vi "ChromaReadReplyMsg.vi"(10 "Boolean_MsgReceiveErr?":bool, 11 "Str_ReplyIn":string) -> (0 "Clu_Result?":T1, 1 "Clu_StepParametersOut":T5, 2 "Str_MsgOut":string, 3 "Enum_ReplyMessage":T6(ring), 4 "Clu_PresetParameterOut":T4, 5 "Clu_RemoteOffsetKeylockResultOut":T2, 6 "Clu_SysSettingOut":T3)   [LabVIEW 2016]
uses:
  TypeDef/Enum_ResultCode.ctl
panel:
  out "BooleanFlag":bool
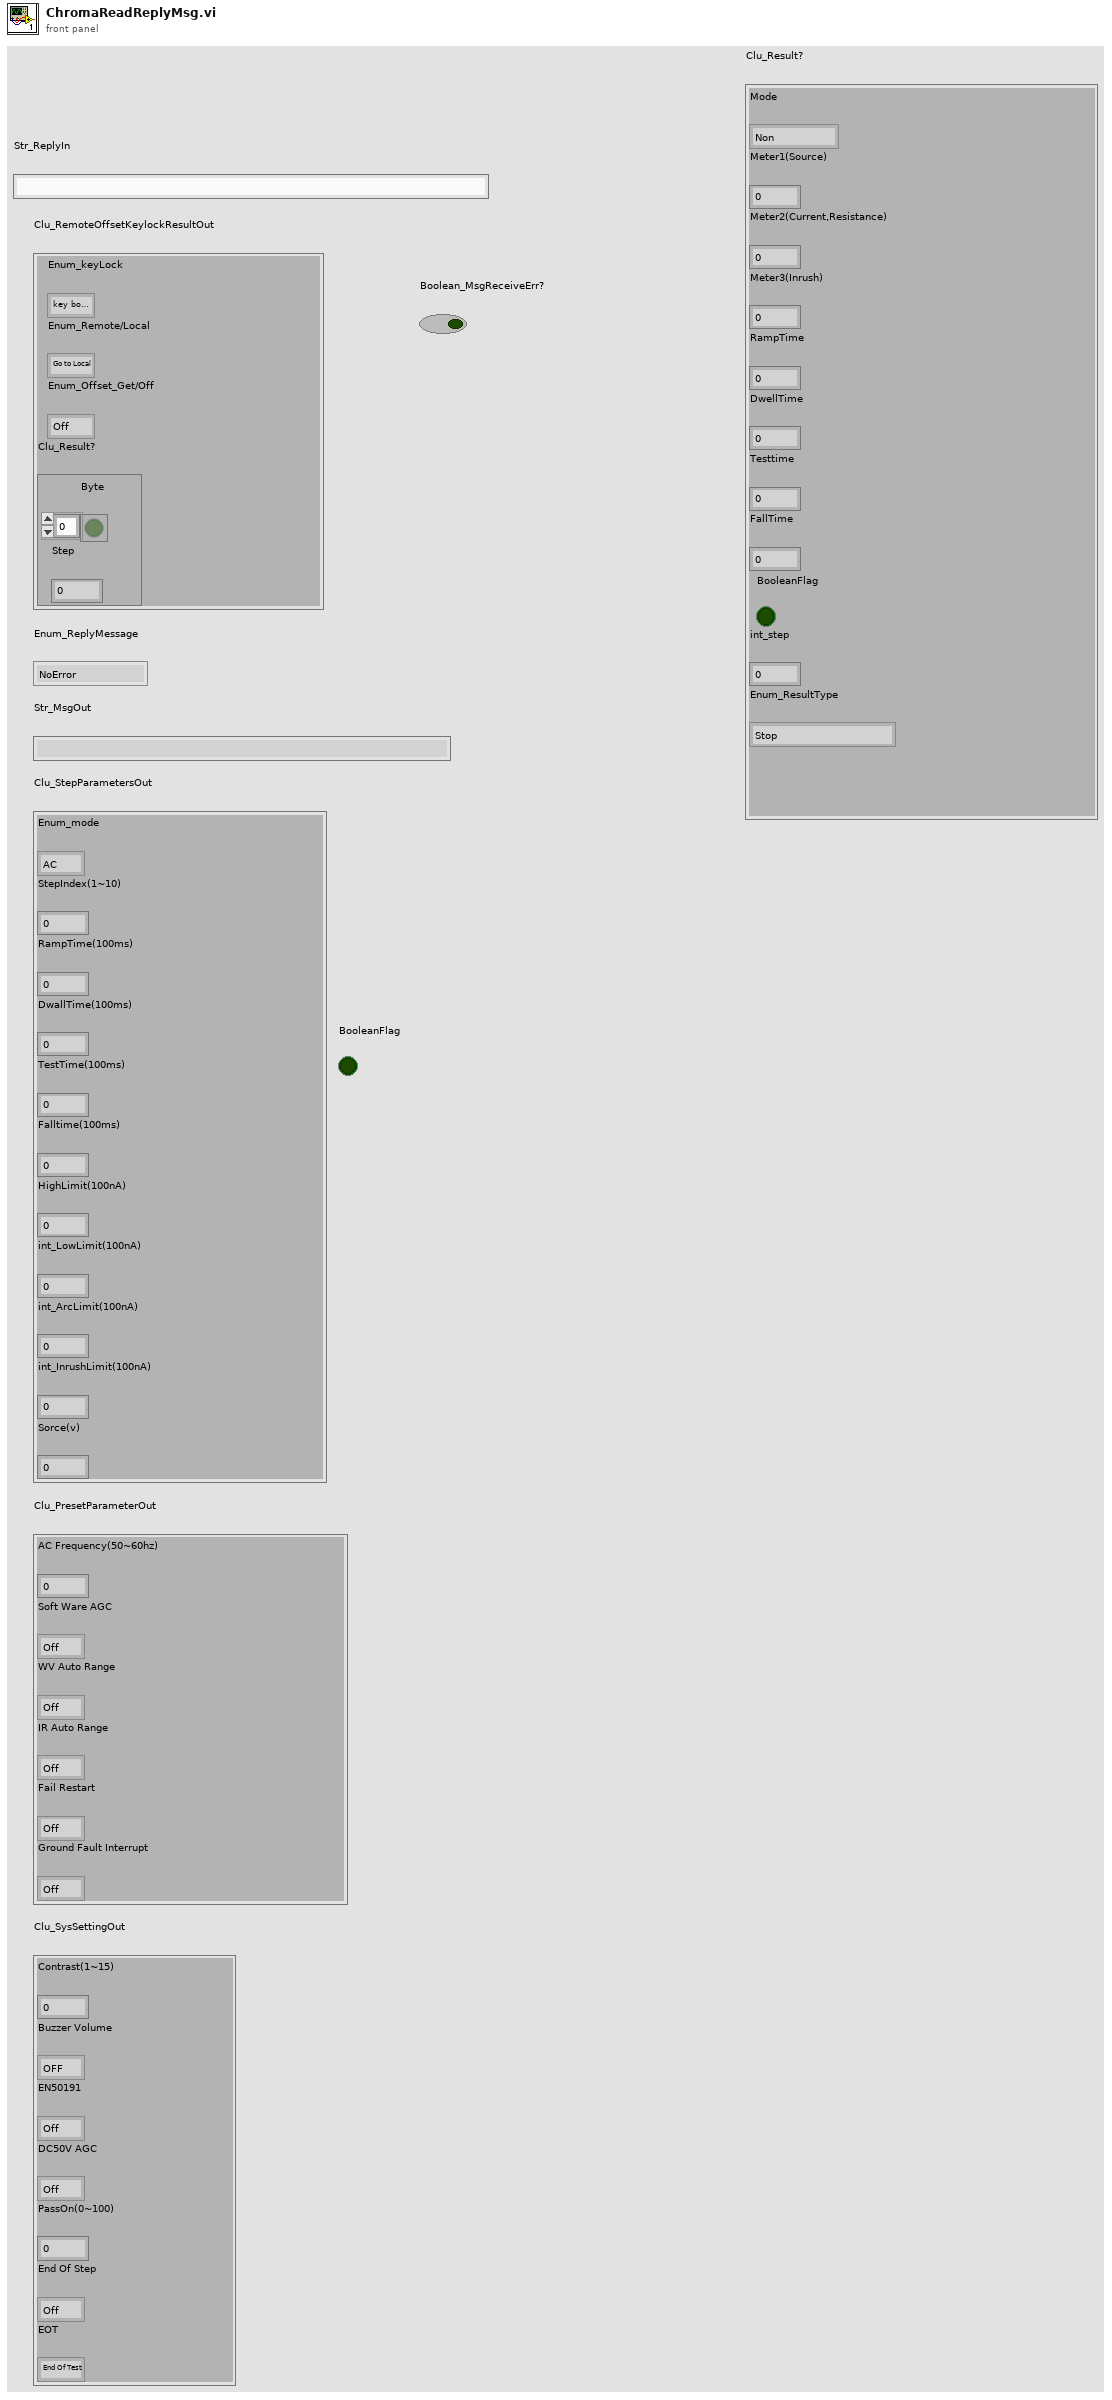
[diagram p1: front panel]
types:
  T1 = cluster{"Mode":enum8{"Non", "AC", "DC", "IR"}, "Meter1(Source)":u16, "Meter2(Current,Resistance)":u32, "Meter3(Inrush)":u32, "RampTime":u16, "DwellTime":u16, "Testtime":u16, "FallTime":u16, "BooleanFlag":bool, "int_step":u8, "Enum_ResultType":enum8{"Stop", "User Interupt", "Can not test", "Testing", "Pass", "Skipped", "GFI Tripped"}}
  T2 = cluster{"Enum_keyLock":enum8{"key board lock Off,recall key lock Off", "key board lock On,recall key lock Off", "key board lock On,recall key lock On"}, "Enum_Remote/Local":enum8{"Go to Local", "Go to Remote", "Go to Remote and Local Lockout"}, "Enum_Offset_Get/Off":enum8{"Off", "Nonuse", "Get"}, "Clu_Result?":cluster{"Byte":bool[], "Step":u8}}
  T3 = cluster{"Contrast(1~15)":u8, "Buzzer Volume":enum8{"OFF", "LOW", "Medium", "High"}, "EN50191":enum8{"Off", "On"}, "DC50V AGC":enum8{"Off", "On"}, "PassOn(0~100)":u8, "End Of Step":enum8{"Off", "On"}, "EOT":enum8{"End Of Test", "End Of Timer"}}
  T4 = cluster{"AC Frequency(50~60hz)":u8, "Soft Ware AGC":enum8{"Off", "On"}, "WV Auto Range":enum8{"Off", "On"}, "IR Auto Range":enum8{"Off", "On"}, "Fail Restart":enum8{"Off", "On"}, "Ground Fault Interrupt":enum8{"Off", "On"}}
  T5 = cluster{"Enum_mode":enum16{"AC", "DC", "IR"}, "StepIndex(1~10)":u8, "RampTime(100ms)":u16, "DwallTime(100ms)":u16, "TestTime(100ms)":u16, "Falltime(100ms)":u16, "HighLimit(100nA)":u32, "int_LowLimit(100nA)":u32, "int_ArcLimit(100nA)":u32, "int_InrushLimit(100nA)":u32, "Sorce(v)":u16}
  T6 = enum16{"NoError", "CommendError", "ParameterError"}
  T7 = enum16{"big-endian, network order", "native, host order", "little-endian"}
  T8 = typedef "Enum_ResultCode.ctl" = enum8{"Stop", "User Interupt", "Can not test", "Testing", "Pass", "Skipped", "GFI Tripped"}
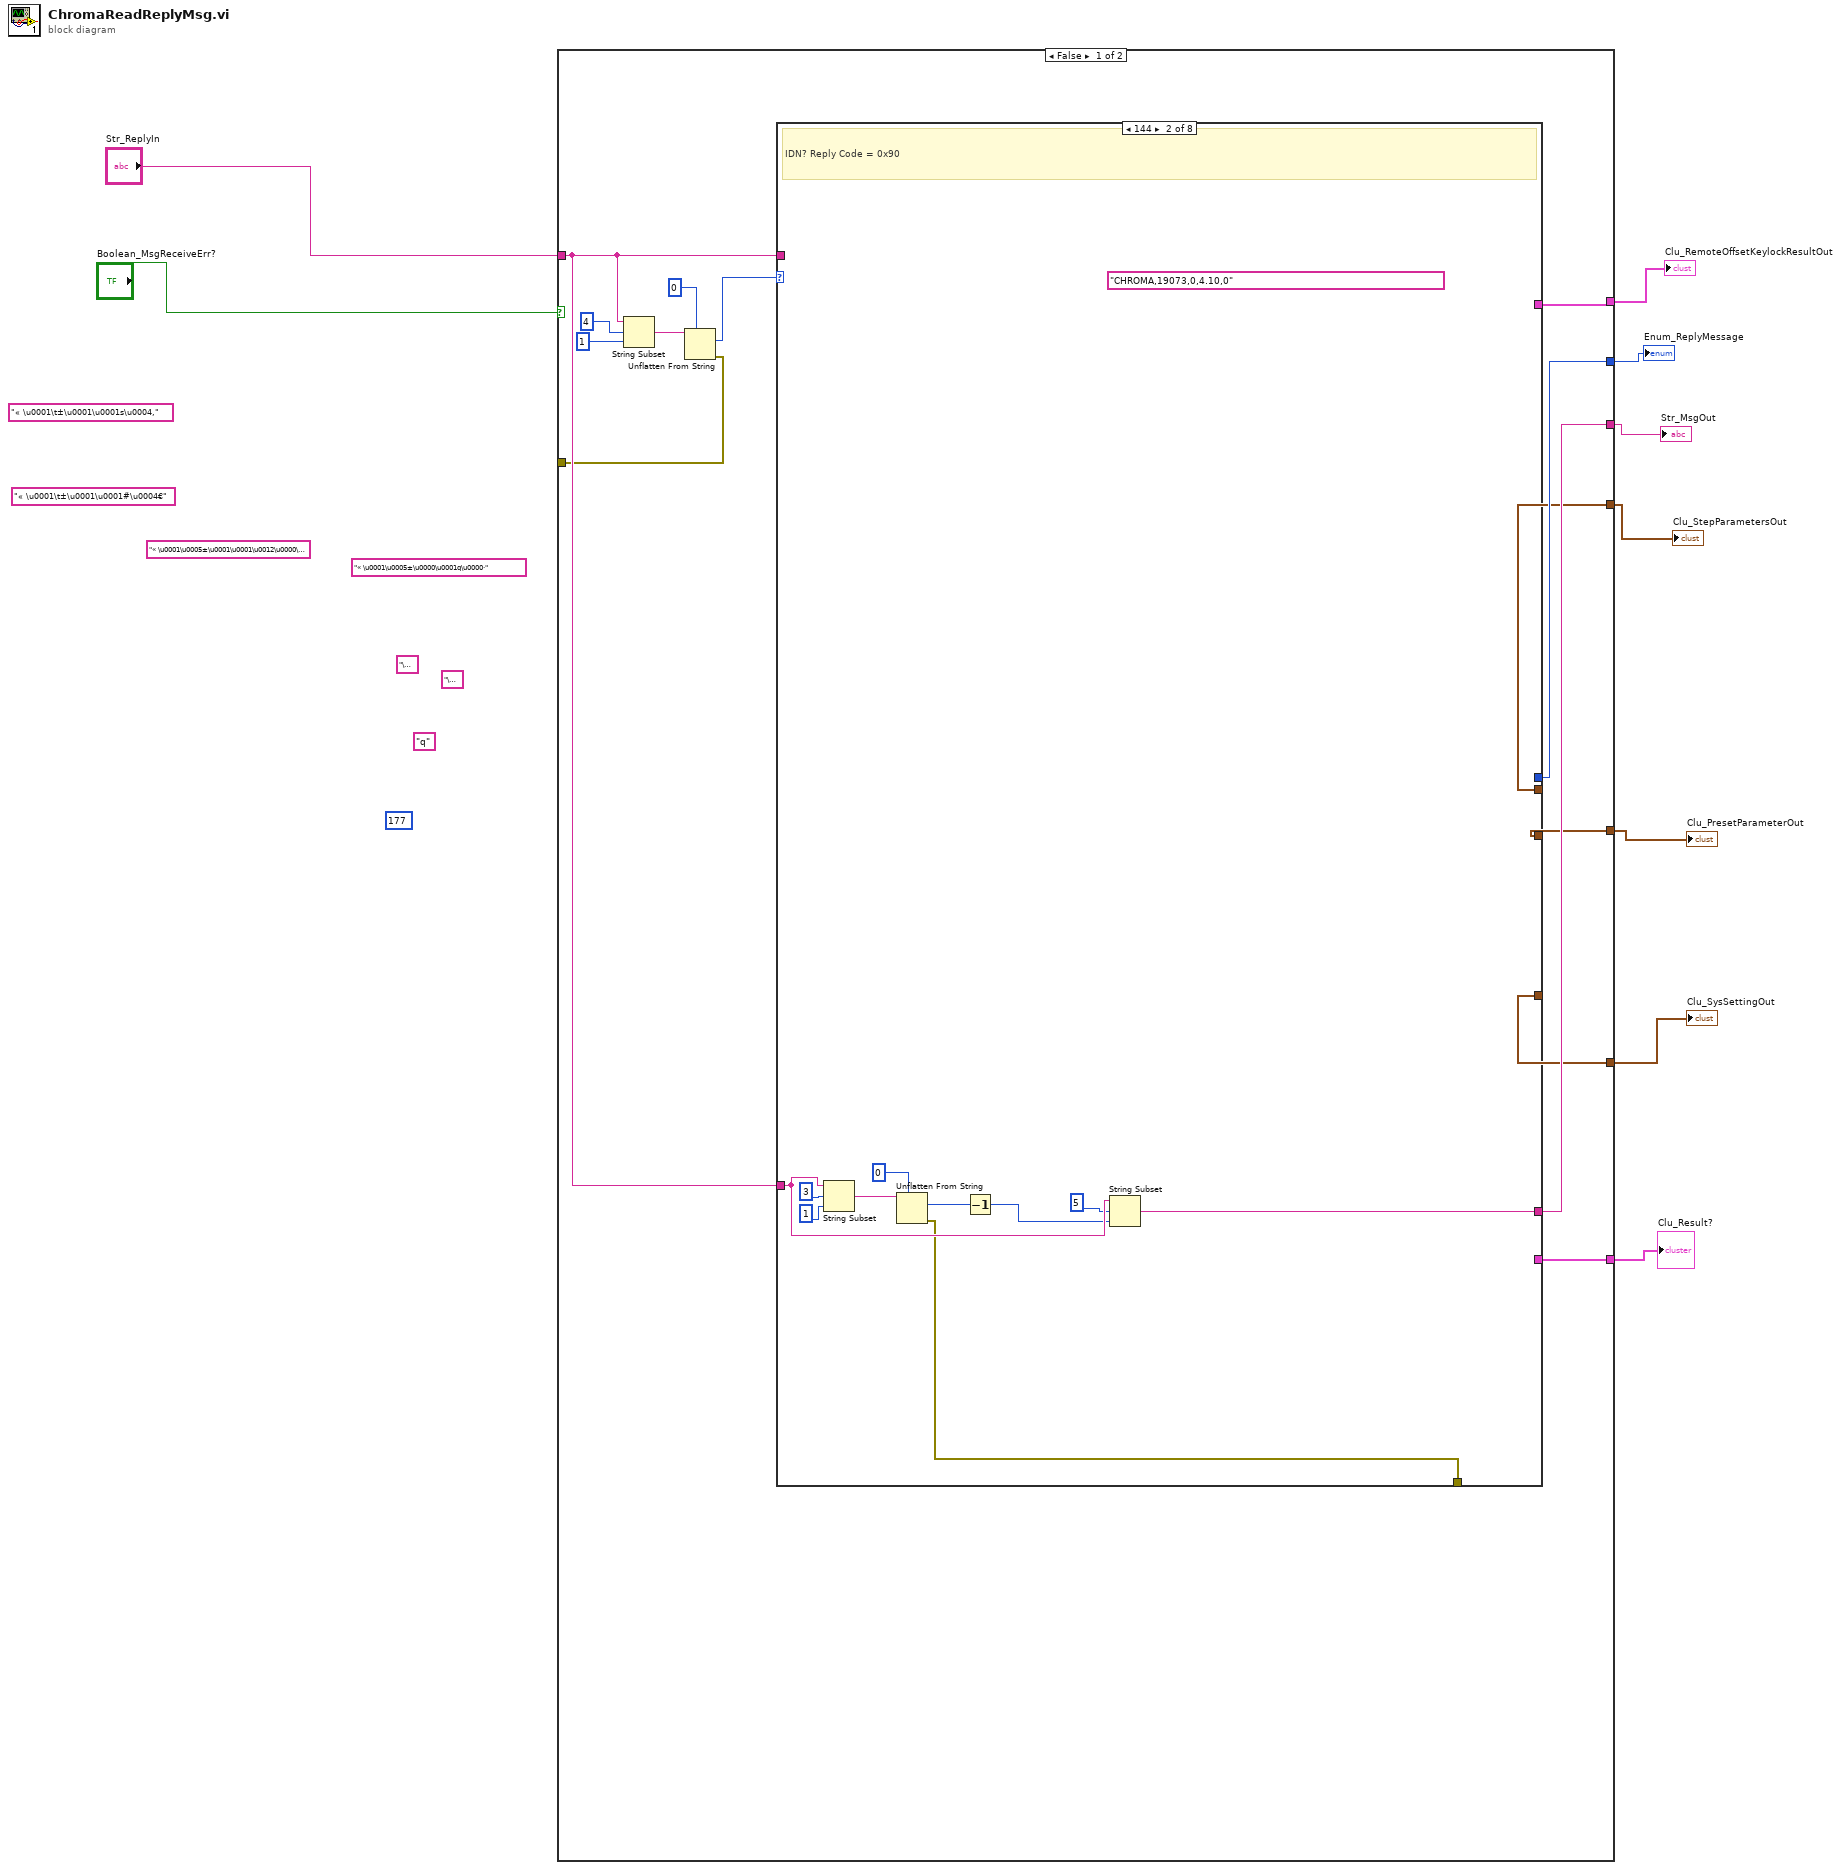
[diagram p0: block diagram]
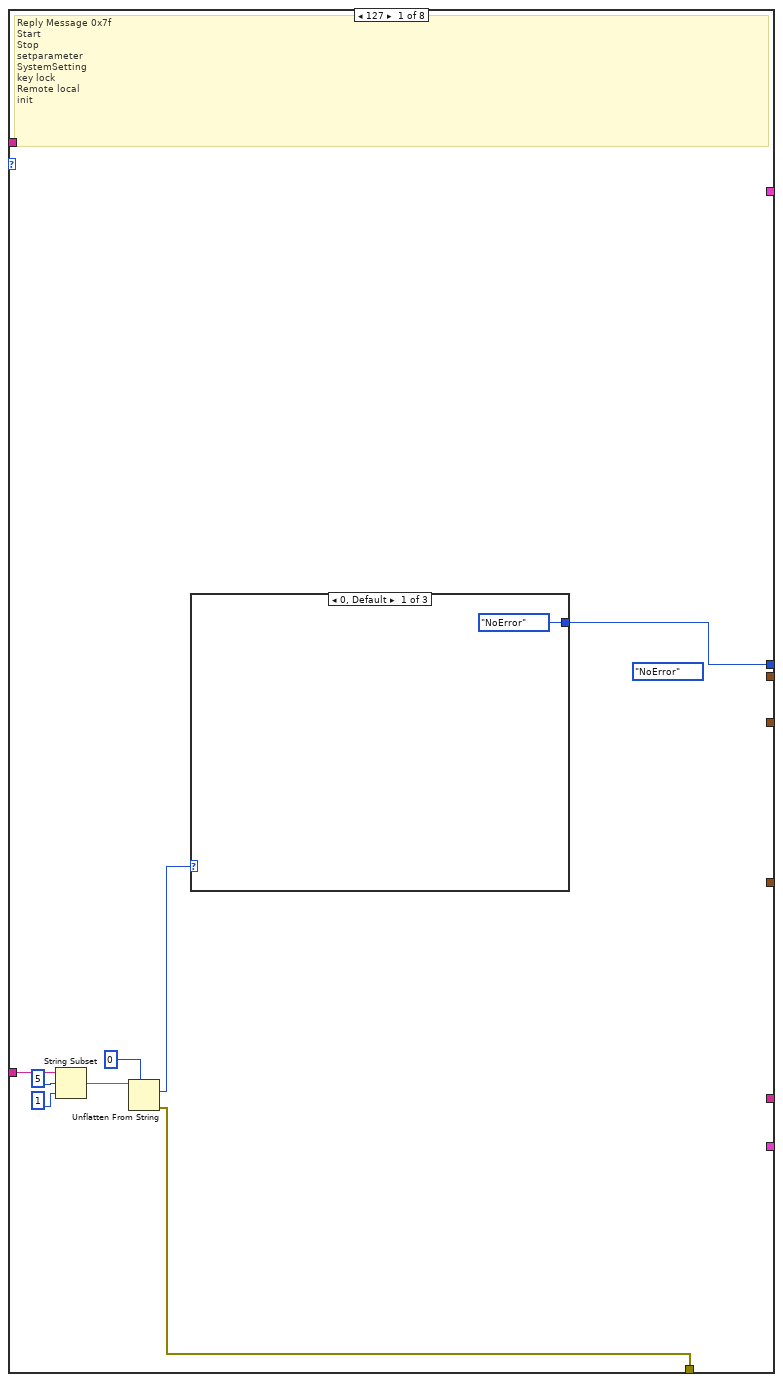
[diagram p2: hidden frame]
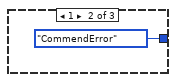
[diagram p3: hidden frame]
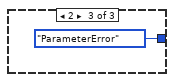
[diagram p4: hidden frame]
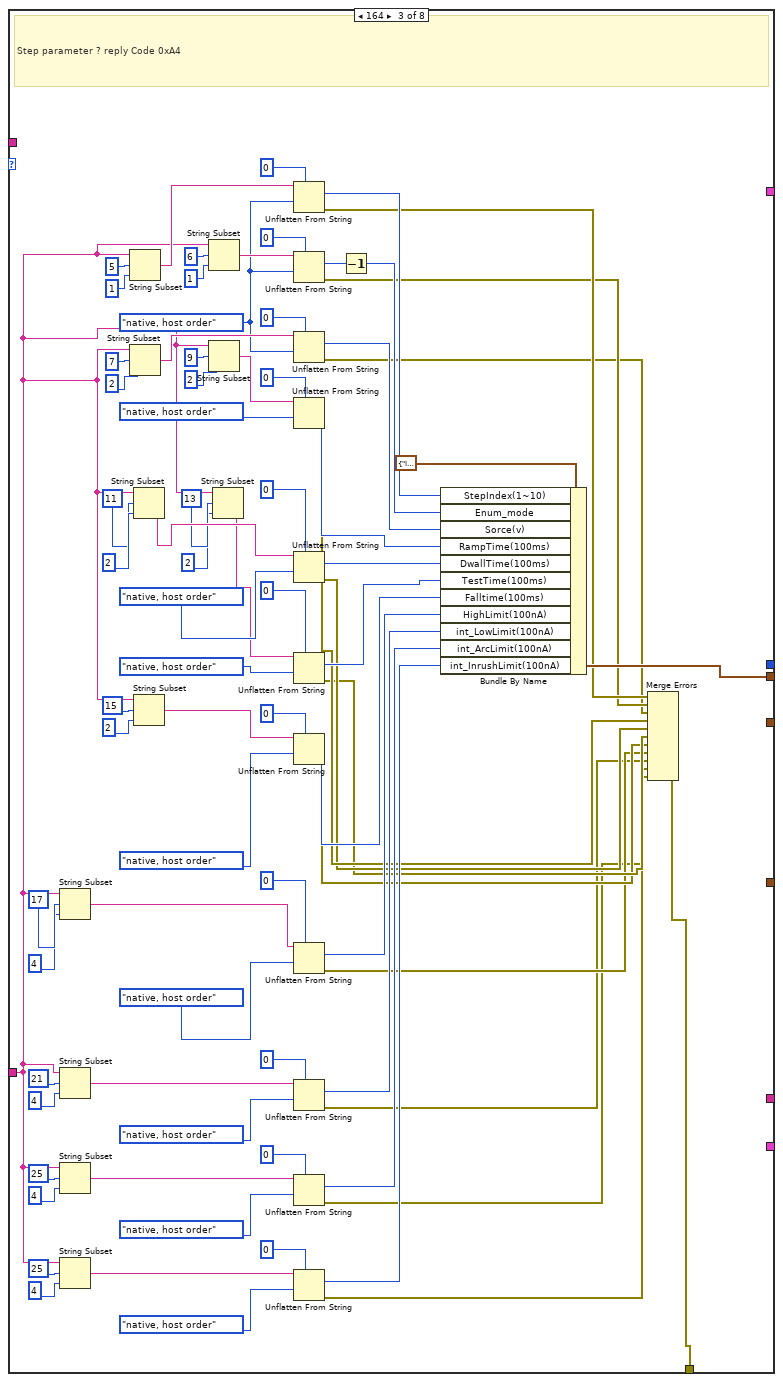
[diagram p5: hidden frame]
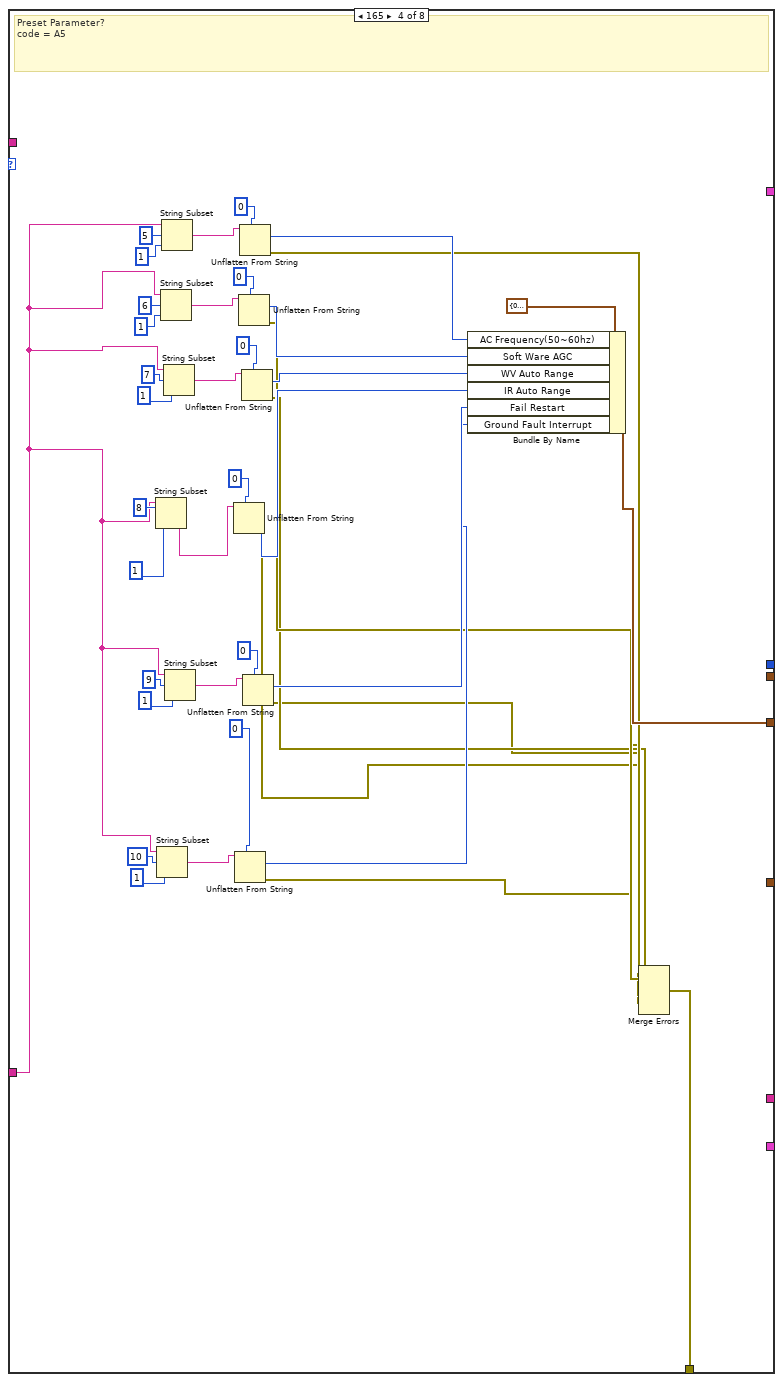
[diagram p6: hidden frame]
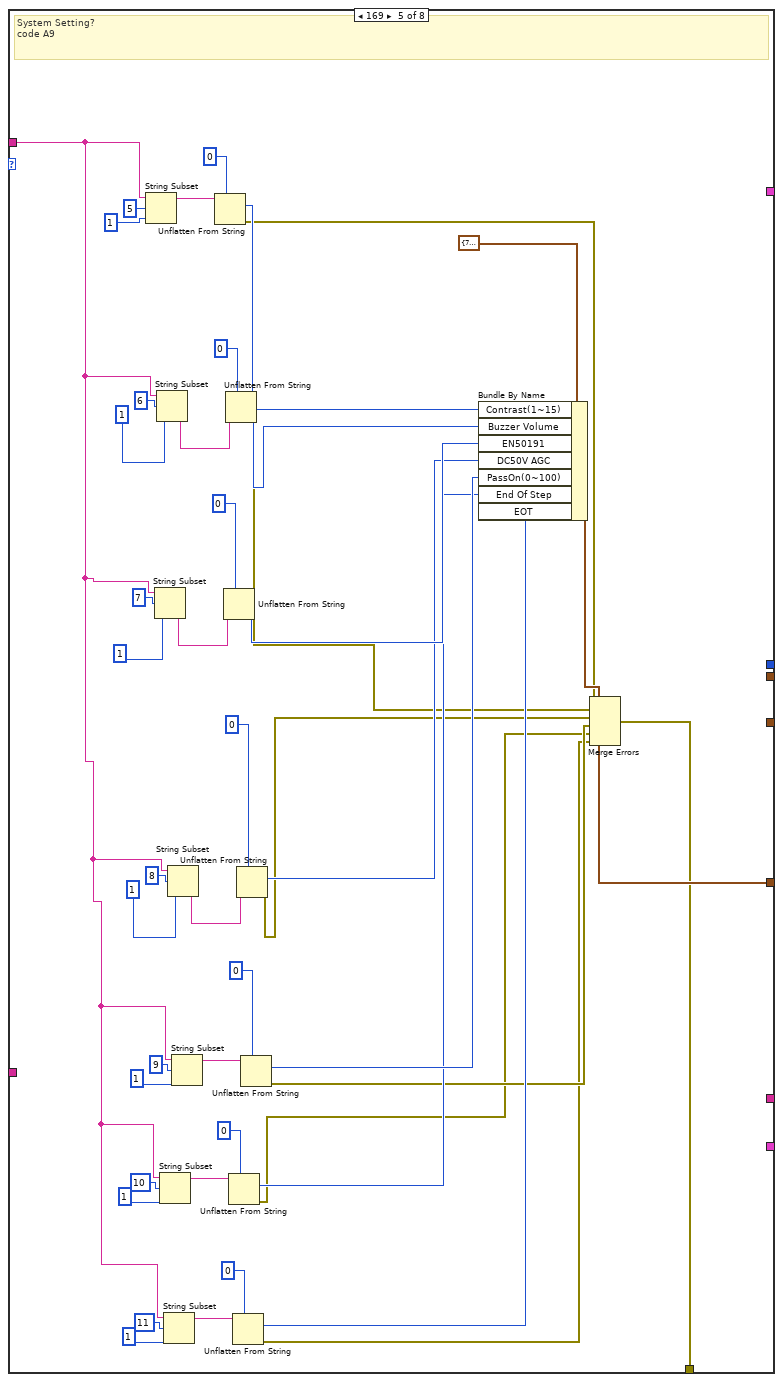
[diagram p7: hidden frame]
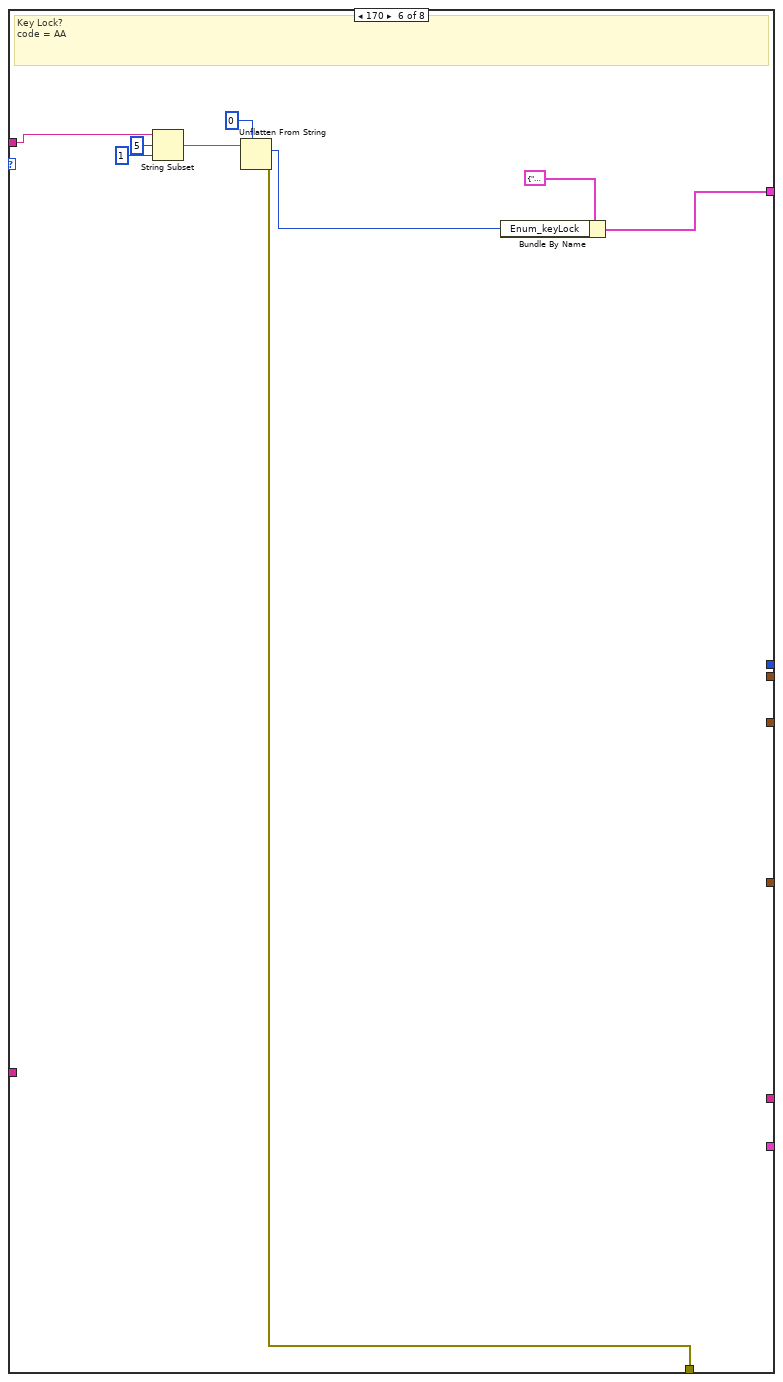
[diagram p8: hidden frame]
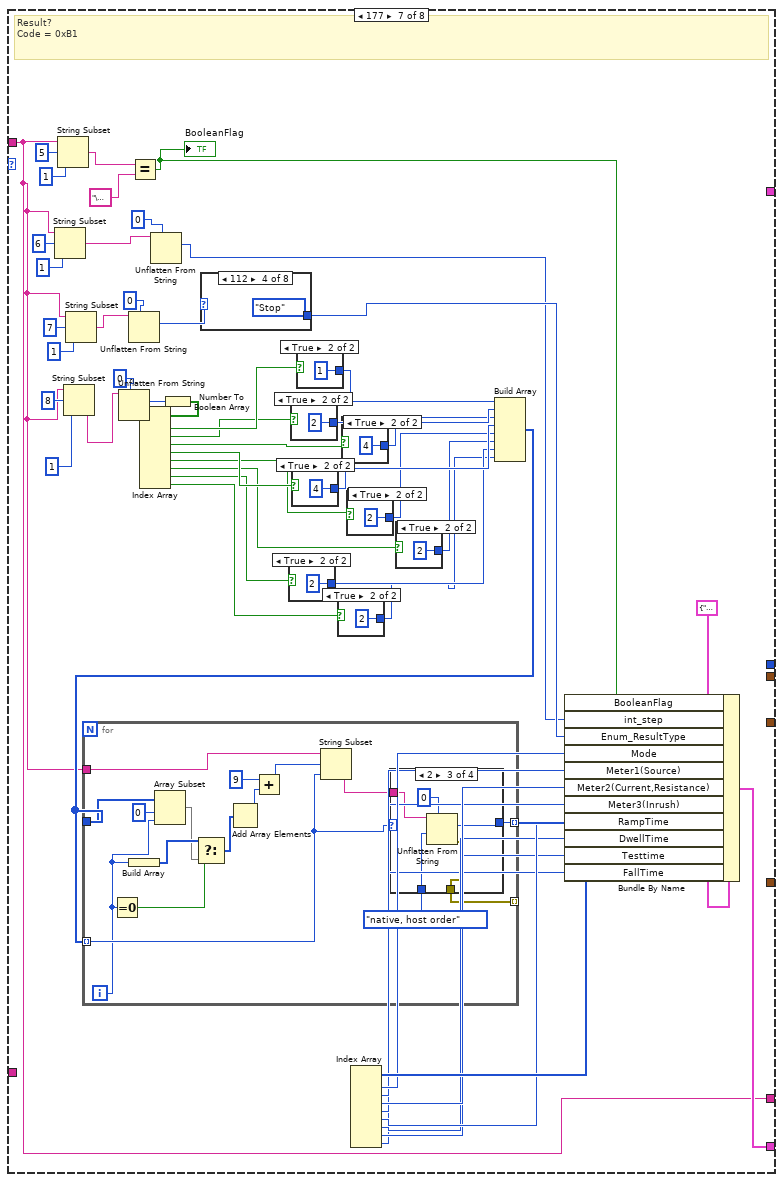
[diagram p9: hidden frame]
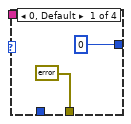
[diagram p10: hidden frame]
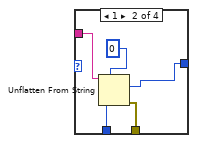
[diagram p11: hidden frame]
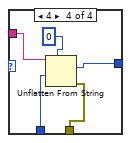
[diagram p12: hidden frame]
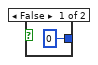
[diagram p13: hidden frame]
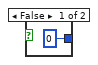
[diagram p14: hidden frame]
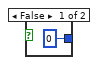
[diagram p15: hidden frame]
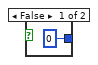
[diagram p16: hidden frame]
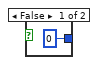
[diagram p17: hidden frame]
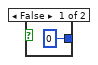
[diagram p18: hidden frame]
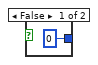
[diagram p19: hidden frame]
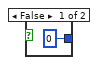
[diagram p20: hidden frame]
diagram:
  (unwired) "« \u0001\t±\u0001\u0001s\u0004," ("Str_ReplyIn 2")
  (unwired) "« \u0001\t±\u0001\u0001#\u0004€" ("Str_ReplyIn 2")
  (unwired) "« \u0001\u0005±\u0001\u0001\u0012\u0000\u0015"
  (unwired) "\u0012"
  (unwired) "q" ("Display")
  (unwired) "\u0000" ("Display")
  (unwired) "« \u0001\u0005±\u0000\u0001q\u0000·" ("Display")
  (unwired) u8 177
  n1 = case shown="False" "Boolean_MsgReceiveErr?" {
    tunnel: "Str_ReplyIn" -> [w13 _]
    tunnel: [w18 _] -> w4
    tunnel: [w17 _] -> w5
    tunnel: [w16 _] -> w6
    tunnel: [w15 _] -> w7
    tunnel: [w14 _] -> w8
    tunnel: [w12 _] -> w9
    tunnel: [w11 _] -> _
    tunnel: [w10 _] -> w1
    frame False {
      n2 = String Subset(string=w13, offset (0)=4, length (rest)=1 ("length (rest)")) -> (substring=w21:string)
      n3 = Unflatten From String(type=u8 0, binary string=w21) -> (value=w19:u8, error out=w11:errorcluster)  [unwired: 3 in, 1 out]
      n4 = case shown="144" w19 {
        tunnel: w13 -> [w31 w40 w62 w139 _ _ _ _]
        tunnel: [w25 _ _ _ _ _ _ _] -> w18
        tunnel: [_ w38 _ _ _ _ w219 _] -> w17
        tunnel: [_ _ w60 _ _ _ _ _] -> w16
        tunnel: [_ _ _ w132 _ _ _ _] -> w15
        tunnel: [_ _ _ _ w209 _ _ _] -> w14
        tunnel: w13 -> [_ _ _ _ w173 w218 w219 _]
        tunnel: [_ _ _ _ _ w211 _ _] -> w12
        tunnel: [w24 w35 w45 w125 w165 w210 _ _] -> _
        tunnel: [_ _ _ _ _ _ w224 _] -> w10
        frame 127 {
          (unwired) T6."NoError"
          # "Reply Message 0x7f\nStart\nStop\nsetparameter\nSystemSetting\nkey lock\nRemote local\ninit"
          n5 = String Subset(string=w31, offset (0)=5, length (rest)=1 ("length (rest)")) -> (substring=w28:string)
          n6 = Unflatten From String(type=u8 0, binary string=w28) -> (value=w26:u8, error out=w24:errorcluster)  [unwired: 3 in, 1 out]
          n7 = case shown="0, Default" w26 {
            tunnel: [T6."NoError" T6."CommendError" T6."ParameterError"] -> w25
            frame 0, Default {
            }
            frame 1 {
            }
            frame 2 {
            }
          }
        }
        frame 144 {
          (unwired) "CHROMA,19073,0,4.10,0"
          # "IDN? Reply Code = 0x90"
          n8 = String Subset(string=w40, offset (0)=3, length (rest)=1 ("length (rest)")) -> (substring=w42:string)
          n9 = Unflatten From String(type=u8 0, binary string=w42) -> (value=w37:u8, error out=w35:errorcluster)  [unwired: 3 in, 1 out]
          n10 = Decrement(x=w37) -> (x-1=w36:u8)
          n11 = String Subset(string=w40, offset (0)=5, length (rest)=w36) -> (substring=w38:string)
        }
        frame 164 {
          w59 = T7."native, host order" ("byte order (0:big-endian, network order)")
          # "Step parameter ? reply Code 0xA4"
          n12 = String Subset(string=w62, offset (0)=17, length (rest)=4 ("length (rest)")) -> (substring=w83:string)
          n13 = String Subset(string=w62, offset (0)=21, length (rest)=4 ("length (rest)")) -> (substring=w78:string)
          n14 = String Subset(string=w62, offset (0)=25, length (rest)=4 ("length (rest)")) -> (substring=w71:string)
          n15 = String Subset(string=w62, offset (0)=25, length (rest)=4 ("length (rest)")) -> (substring=w65:string)
          n16 = String Subset(string=w62, offset (0)=5, length (rest)=1 ("length (rest)")) -> (substring=w122:string)
          n17 = String Subset(string=w62, offset (0)=7, length (rest)=2 ("length (rest)")) -> (substring=w112:string)
          n18 = String Subset(string=w62, offset (0)=11, length (rest)=2 ("length (rest)")) -> (substring=w101:string)
          n19 = String Subset(string=w62, offset (0)=15, length (rest)=2 ("length (rest)")) -> (substring=w89:string)
          n20 = String Subset(string=w62, offset (0)=6, length (rest)=1 ("length (rest)")) -> (substring=w115:string)
          n21 = String Subset(string=w62, offset (0)=9, length (rest)=2 ("length (rest)")) -> (substring=w107:string)
          n22 = String Subset(string=w62, offset (0)=13, length (rest)=2 ("length (rest)")) -> (substring=w95:string)
          n23 = Unflatten From String(type=u8 0 ("Step"), binary string=w122, byte order (0:big-endian, network order)=w59) -> (value=w119:u8, error out=w56:errorcluster)  [unwired: 2 in, 1 out]
          n24 = Unflatten From String(type=u8 0, binary string=w115, byte order (0:big-endian, network order)=w59) -> (value=w58:u8, error out=w55:errorcluster)  [unwired: 2 in, 1 out]
          n25 = Unflatten From String(type=u16 0, binary string=w112, byte order (0:big-endian, network order)=w59) -> (value=w110:u16, error out=w54:errorcluster)  [unwired: 2 in, 1 out]
          n26 = Unflatten From String(type=u16 0, binary string=w107, byte order (0:big-endian, network order)=T7."native, host order") -> (value=w104:u16, error out=w53:errorcluster)  [unwired: 2 in, 1 out]
          n27 = Unflatten From String(type=u16 0, binary string=w101, byte order (0:big-endian, network order)=T7."native, host order") -> (value=w98:u16, error out=w52:errorcluster)  [unwired: 2 in, 1 out]
          n28 = Unflatten From String(type=u16 0, binary string=w95, byte order (0:big-endian, network order)=T7."native, host order") -> (value=w92:u16, error out=w51:errorcluster)  [unwired: 2 in, 1 out]
          n29 = Unflatten From String(type=u16 0, binary string=w89, byte order (0:big-endian, network order)=T7."native, host order") -> (value=w86:u16, error out=w50:errorcluster)  [unwired: 2 in, 1 out]
          n30 = Unflatten From String(type=u32 0, binary string=w83, byte order (0:big-endian, network order)=T7."native, host order") -> (value=w80:u32, error out=w49:errorcluster)  [unwired: 2 in, 1 out]
          n31 = Unflatten From String(type=u32 0, binary string=w78, byte order (0:big-endian, network order)=T7."native, host order") -> (value=w74:u32, error out=w48:errorcluster)  [unwired: 2 in, 1 out]
          n32 = Unflatten From String(type=u32 0, binary string=w71, byte order (0:big-endian, network order)=T7."native, host order") -> (value=w68:u32, error out=w47:errorcluster)  [unwired: 2 in, 1 out]
          n33 = Unflatten From String(type=u32 0, binary string=w65, byte order (0:big-endian, network order)=T7."native, host order") -> (value=w61:u32, error out=w46:errorcluster)  [unwired: 2 in, 1 out]
          n34 = Decrement(x=w58) -> (x-1=w57:u8)
          n35 = Bundle By Name(cluster=T5 {"Enum_mode"=enum."IR", "StepIndex(1~10)"=1, "RampTime(100ms)"=20, "DwallTime(100ms)"=0, "TestTime(100ms)"=50, "Falltime(100ms)"=30, "HighLimit(100nA)"=10000, "int_LowLimit(100nA)"=1000, "int_ArcLimit(100nA)"=10000, "int_InrushLimit(100nA)"=0, "Sorce(v)"=1000} ("Clu_StepParameters"), "StepIndex(1~10)"=w119, "Enum_mode"=w57, "Sorce(v)"=w110, "RampTime(100ms)"=w104, "DwallTime(100ms)"=w98, "TestTime(100ms)"=w92, "Falltime(100ms)"=w86, "HighLimit(100nA)"=w80, "int_LowLimit(100nA)"=w74, "int_ArcLimit(100nA)"=w68, "int_InrushLimit(100nA)"=w61) -> (w60:T5)
          n36 = Merge Errors(w56, w55, w54, w53, w52, w51, w50, w49, w48, w47, w46) -> (w45:errorcluster)
        }
        frame 165 {
          # "Preset Parameter?\ncode = A5"
          n37 = String Subset(string=w139, offset (0)=8, length (rest)=1 ("length (rest)")) -> (substring=w148:string)
          n38 = String Subset(string=w139, offset (0)=10, length (rest)=1 ("length (rest)")) -> (substring=w140:string)
          n39 = String Subset(string=w139, offset (0)=6, length (rest)=1 ("length (rest)")) -> (substring=w156:string)
          n40 = String Subset(string=w139, offset (0)=5, length (rest)=1 ("length (rest)")) -> (substring=w163:string)
          n41 = String Subset(string=w139, offset (0)=7, length (rest)=1 ("length (rest)")) -> (substring=w155:string)
          n42 = String Subset(string=w139, offset (0)=9, length (rest)=1 ("length (rest)")) -> (substring=w147:string)
          n43 = Unflatten From String(type=u8 0, binary string=w148) -> (value=w135:u8, error out=w128:errorcluster)  [unwired: 3 in, 1 out]
          n44 = Unflatten From String(type=u8 0, binary string=w140) -> (value=w133:u8, error out=w126:errorcluster)  [unwired: 3 in, 1 out]
          n45 = Unflatten From String(type=u8 0, binary string=w156) -> (value=w137:u8, error out=w130:errorcluster)  [unwired: 3 in, 1 out]
          n46 = Unflatten From String(type=u8 0, binary string=w163) -> (value=w138:u8, error out=w131:errorcluster)  [unwired: 3 in, 1 out]
          n47 = Unflatten From String(type=u8 0, binary string=w155) -> (value=w136:u8, error out=w129:errorcluster)  [unwired: 3 in, 1 out]
          n48 = Unflatten From String(type=u8 0, binary string=w147) -> (value=w134:u8, error out=w127:errorcluster)  [unwired: 3 in, 1 out]
          n49 = Bundle By Name(cluster=T4 {"AC Frequency(50~60hz)"=0, "Soft Ware AGC"=enum."Off", "WV Auto Range"=enum."Off", "IR Auto Range"=enum."Off", "Fail Restart"=enum."Off", "Ground Fault Interrupt"=enum."Off"} ("Clu_PresetParameter"), "AC Frequency(50~60hz)"=w138, "Soft Ware AGC"=w137, "WV Auto Range"=w136, "IR Auto Range"=w135, "Fail Restart"=w134, "Ground Fault Interrupt"=w133) -> (w132:T4)
          n50 = Merge Errors(w131, w130, w129, w128, w127, w126) -> (w125:errorcluster)
        }
        frame 169 {
          # "System Setting?\ncode A9"
          n51 = String Subset(string=w173, offset (0)=5, length (rest)=1 ("length (rest)")) -> (substring=w206:string)
          n52 = String Subset(string=w173, offset (0)=7, length (rest)=1 ("length (rest)")) -> (substring=w196:string)
          n53 = String Subset(string=w173, offset (0)=6, length (rest)=1 ("length (rest)")) -> (substring=w202:string)
          n54 = String Subset(string=w173, offset (0)=10, length (rest)=1 ("length (rest)")) -> (substring=w181:string)
          n55 = String Subset(string=w173, offset (0)=11, length (rest)=1 ("length (rest)")) -> (substring=w176:string)
          n56 = String Subset(string=w173, offset (0)=8, length (rest)=1 ("length (rest)")) -> (substring=w192:string)
          n57 = String Subset(string=w173, offset (0)=9, length (rest)=1 ("length (rest)")) -> (substring=w185:string)
          n58 = Unflatten From String(type=u8 0, binary string=w206) -> (value=w204:u8, error out=w171:errorcluster)  [unwired: 3 in, 1 out]
          n59 = Unflatten From String(type=u8 0, binary string=w196) -> (value=w194:u8)  [unwired: 3 in, 2 out]
          n60 = Unflatten From String(type=u8 0, binary string=w202) -> (value=w199:u8, error out=w170:errorcluster)  [unwired: 3 in, 1 out]
          n61 = Unflatten From String(type=u8 0, binary string=w181) -> (value=w178:u8, error out=w167:errorcluster)  [unwired: 3 in, 1 out]
          n62 = Unflatten From String(type=u8 0, binary string=w176) -> (value=w172:u8, error out=w166:errorcluster)  [unwired: 3 in, 1 out]
          n63 = Unflatten From String(type=u8 0, binary string=w192) -> (value=w189:u8, error out=w169:errorcluster)  [unwired: 3 in, 1 out]
          n64 = Unflatten From String(type=u8 0, binary string=w185) -> (value=w183:u8, error out=w168:errorcluster)  [unwired: 3 in, 1 out]
          n65 = Bundle By Name(cluster=T3 {"Contrast(1~15)"=7, "Buzzer Volume"=enum."High", "EN50191"=enum."Off", "DC50V AGC"=enum."On", "PassOn(0~100)"=0, "End Of Step"=enum."Off", "EOT"=enum."End Of Test"} ("Clu_SysSetting"), "Contrast(1~15)"=w204, "Buzzer Volume"=w199, "EN50191"=w194, "DC50V AGC"=w189, "PassOn(0~100)"=w183, "End Of Step"=w178, "EOT"=w172) -> (w209:T3)
          n66 = Merge Errors(w171, w170, w169, w168, w167, w166) -> (w165:errorcluster)
        }
        frame 170 {
          # "Key Lock?\ncode = AA"
          n67 = String Subset(string=w218, offset (0)=5, length (rest)=1 ("length (rest)")) -> (substring=w215:string)
          n68 = Unflatten From String(type=u8 0, binary string=w215) -> (value=w212:u8, error out=w210:errorcluster)  [unwired: 3 in, 1 out]
          n69 = Bundle By Name(cluster=T2 {"Enum_keyLock"=enum."key board lock Off,recall key lock Off", "Enum_Remote/Local"=enum."Go to Local", "Enum_Offset_Get/Off"=enum."Off", "Clu_Result?"={"Byte"=[FALSE, FALSE, FALSE, FALSE, FALSE, FALSE, FALSE, FALSE], "Step"=0}} ("Clu_RemoteOffsetKeylockResult"), "Enum_keyLock"=w212) -> (w211:T2)
        }
        frame 177 {
          # "Result?\nCode = 0xB1"
          n70 = String Subset(string=w219, offset (0)=6, length (rest)=1 ("length (rest)")) -> (substring=w263:string)
          n71 = String Subset(string=w219, offset (0)=5, length (rest)=1 ("length (rest)")) -> (substring=w267:string)
          n72 = String Subset(string=w219, offset (0)=8, length (rest)=1 ("length (rest)")) -> (substring=w253:string)
          n73 = String Subset(string=w219, offset (0)=7, length (rest)=1 ("length (rest)")) -> (substring=w258:string)
          n74 = Unflatten From String(type=u8 0, binary string=w253) -> (value=w252:u8)  [unwired: 3 in, 2 out]
          n75 = Unflatten From String(type=u8 0, binary string=w258) -> (value=w257:u8)  [unwired: 3 in, 2 out]
          n76 = Equal?(x=w267, y="\u0001") -> (x = y?=w220:bool)
          "BooleanFlag" <- w220
          n77 = Unflatten From String(type=u8 0, binary string=w263) -> (value=w221:u8)  [unwired: 3 in, 2 out]
          n78 = Number To Boolean Array(number=w252) -> (Boolean array=w251:bool[])
          n79 = Index Array(array=w251) -> (element #1=w250:bool, element #2=w249:bool, element #3=w248:bool, element #4=w247:bool, element #5=w246:bool, element #6=w245:bool, element #7=w244:bool, element #8=w243:bool)  [unwired: 8 in]
          n80 = case shown="112" w257 {
            tunnel: [Enum_ResultCode."Can not test" ("Enum_ResultType") Enum_ResultCode."User Interupt" ("Enum_ResultType") Enum_ResultCode."Skipped" ("Enum_ResultType") Enum_ResultCode."Stop" ("Enum_ResultType") Enum_ResultCode."Pass" ("Enum_ResultType") Enum_ResultCode."Skipped" ("Enum_ResultType") Enum_ResultCode."Pass" ("Enum_ResultType") Enum_ResultCode."Testing" ("Enum_ResultType")] -> w222
            frame 114 {
            }
            frame 113 {
            }
            frame 0, Default {
            }
            frame 112 {
            }
            frame 116 {
            }
            frame 117 {
            }
            frame 121 {
            }
            frame 115 {
            }
          }
          n81 = case shown="True" w244 {
            tunnel: [0 2] -> w236
            frame False {
            }
            frame True {
            }
          }
          n82 = case shown="True" w249 {
            tunnel: [0 2] -> w241
            frame False {
            }
            frame True {
            }
          }
          n83 = case shown="True" w247 {
            tunnel: [0 4] -> w239
            frame False {
            }
            frame True {
            }
          }
          n84 = case shown="True" w250 {
            tunnel: [0 1] -> w242
            frame False {
            }
            frame True {
            }
          }
          n85 = case shown="True" w243 {
            tunnel: [0 2] -> w235
            frame False {
            }
            frame True {
            }
          }
          n86 = case shown="True" w248 {
            tunnel: [0 4] -> w240
            frame False {
            }
            frame True {
            }
          }
          n87 = case shown="True" w246 {
            tunnel: [0 2] -> w238
            frame False {
            }
            frame True {
            }
          }
          n88 = case shown="True" w245 {
            tunnel: [0 2] -> w237
            frame False {
            }
            frame True {
            }
          }
          n89 = Build Array(w242, w241, w240, w239, w238, w237, w236, w235) -> (w234:i32[])
          n90 = for {
            tunnel: w234 -> [w277] mode=indexing
            tunnel: w234 -> [w285]
            tunnel: w219 -> [w282]
            tunnel: [w280] -> _ mode=indexing
            tunnel: [w276] -> w233 mode=indexing
            i -> [w274]
            n91 = Equal To 0?(x=w274) -> (x = 0?=w275:bool)
            n92 = Build Array(w274) -> (w273:i32[])
            n93 = Array Subset(array=w285, index=0, length=w274) -> (w272:i32[])
            n94 = Select(t=w273, s=w275, f=w272) -> (s? t:f=w271:i32[])
            n95 = Add Array Elements(numeric array=w271) -> (sum=w284:i32)
            n96 = Add(x=9, y=w284) -> (x+y=w281:i32)
            n97 = String Subset(string=w282, offset (0)=w281, length (rest)=w277) -> (substring=w279:string)
            n98 = case shown="2" w277 {
              tunnel: [errorcluster {"status"=FALSE, "code"=0, "source"=""} ("error constant") w292 w295 w300] -> w280
              tunnel: w279 -> [_ w291 w297 w302]
              tunnel: T7."native, host order" ("byte order (0:big-endian, network order)") -> [_ w290 w296 w301]
              tunnel: [u32 0 w288 w293 w299] -> w276
              frame 0, Default {
              }
              frame 1 {
                n99 = Unflatten From String(type=u8 0, binary string=w291, byte order (0:big-endian, network order)=w290) -> (value=w288:u8, error out=w292:errorcluster)  [unwired: 2 in, 1 out]
              }
              frame 2 {
                n100 = Unflatten From String(type=u16 0, binary string=w297, byte order (0:big-endian, network order)=w296) -> (value=w293:u16, error out=w295:errorcluster)  [unwired: 2 in, 1 out]
              }
              frame 4 {
                n101 = Unflatten From String(type=u32 0, binary string=w302, byte order (0:big-endian, network order)=w301) -> (value=w299:u32, error out=w300:errorcluster)  [unwired: 2 in, 1 out]
              }
            }
          }
          n102 = Index Array(array=w233) -> (element #1=w232:u32, element #2=w231:u32, element #3=w230:u32, element #4=w229:u32, element #5=w228:u32, element #6=w227:u32, element #7=w226:u32, element #8=w225:u32)  [unwired: 8 in]
          n103 = Bundle By Name(cluster=T1 {"Mode"=enum."Non", "Meter1(Source)"=0, "Meter2(Current,Resistance)"=0, "Meter3(Inrush)"=0, "RampTime"=0, "DwellTime"=0, "Testtime"=0, "FallTime"=0, "BooleanFlag"=FALSE, "int_step"=0, "Enum_ResultType"=enum."Skipped"}, "BooleanFlag"=w220, "int_step"=w221, "Enum_ResultType"=w222, "Mode"=w232, "Meter1(Source)"=w231, "Meter2(Current,Resistance)"=w230, "Meter3(Inrush)"=w229, "RampTime"=w228, "DwellTime"=w227, "Testtime"=w226, "FallTime"=w225) -> (w224:T1)
        }
        frame Default {
        }
      }
    }
    frame True {
    }
  }
  "Enum_ReplyMessage" <- w4
  "Str_MsgOut" <- w5
  "Clu_StepParametersOut" <- w6
  "Clu_PresetParameterOut" <- w7
  "Clu_SysSettingOut" <- w8
  "Clu_RemoteOffsetKeylockResultOut" <- w9
  "Clu_Result?" <- w1
